vi "zadanie2pawelprokopiuk.vi"() -> ()   [LabVIEW 2021]
panel:
  out "min temp":dbl
  out "max temp":dbl
  in  "URL":string="dstp://10.42.14.239/temperatura"
  out "Temperatura":T1(graph)
  in  "stop":bool
  in  "Zapis do pliku":bool
  in  "prog dolny":dbl
  in  "prog gorny":dbl=25.8
  out "alarm dolny":bool
  out "alarm gorny":bool
  out "T chwilowa":dbl
  out "T srednia":dbl
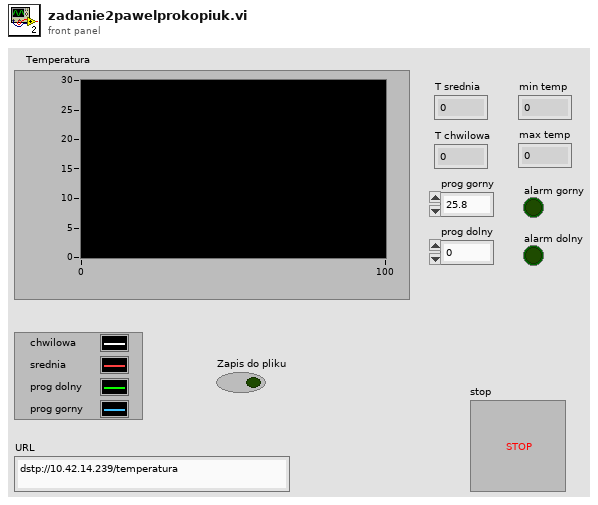
[diagram p1: front panel]
types:
  T1 = cluster{dbl, dbl, "Próg dolny":dbl, "Próg górny":dbl}
  T2 = enum16{"Read", "Write", "ReadWrite", "BufferedRead", "BufferedReadWrite"}
  T3 = enum16{"open", "replace", "create", "open or create", "replace or create", "replace or create with confirmation"}
  T4 = cluster{dbl, dbl, "prog dolny":dbl, "prog gorny":dbl}
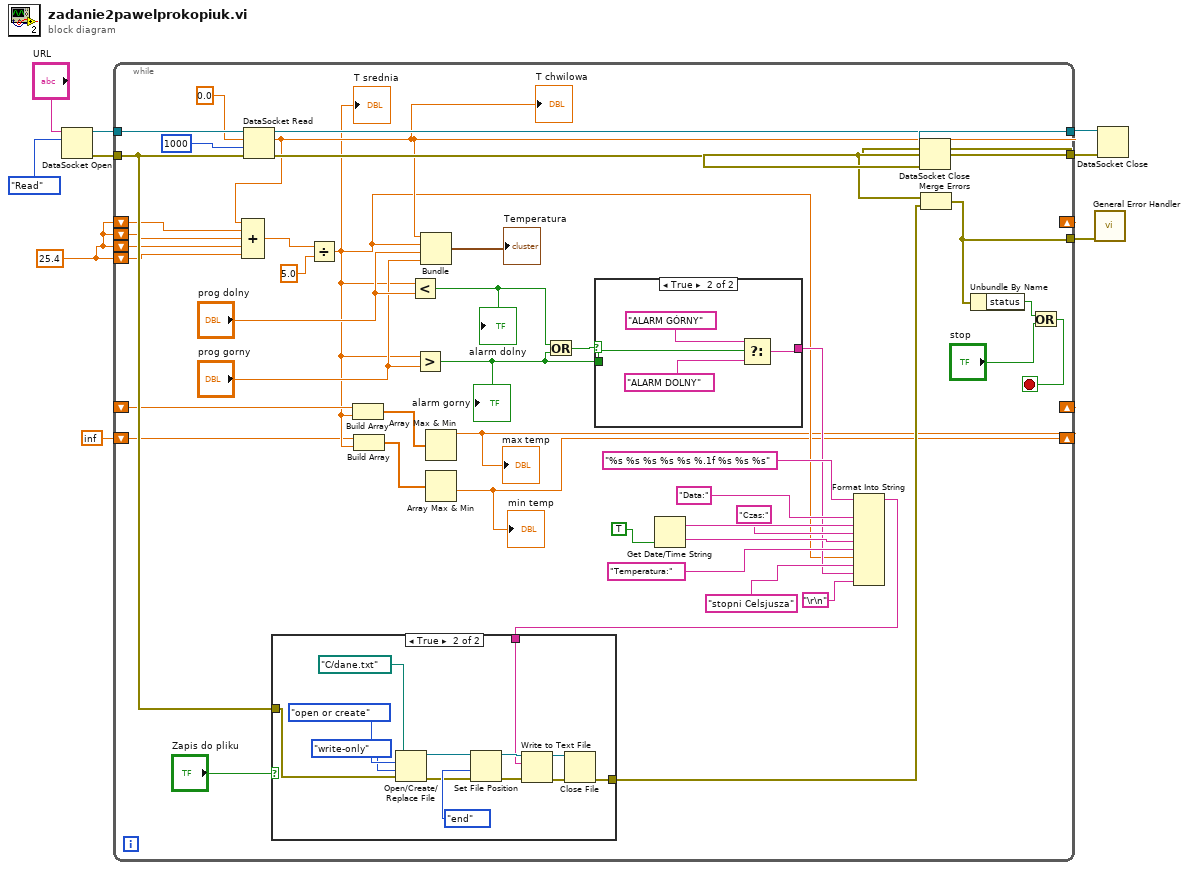
[diagram p0: block diagram]
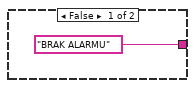
[diagram p2: hidden frame]
diagram:
  w2 = 25.4
  n1 = DataSocket Open(10:T2."Read" ("mode"), 11:"URL") -> (0:w8:errorcluster, 3:w9:refnum<k13>)  [unwired: 2 in]
  n2 = while {
    tunnel: w9 -> [w51]
    tunnel: [w50] -> w4
    tunnel: w8 -> [w44]
    tunnel: [w23] -> w3
    tunnel: [w42] -> w6
    shift-right: [w18] -> _
    shift-left: w2 -> [w22]
    shift-left: w2 -> [w21]
    shift-left: w2 -> [w20]
    shift-left: w2 -> [w19]
    shift-right: [w12] -> _
    shift-left: _ -> [w16]
    shift-right: [w11] -> _
    shift-left: inf -> [w14]
    stop <- w48 stop-if-true
    n3 = DataSocket Read(8:w44, 9:1000, 10:0.0, 11:w51) -> (0:w23:errorcluster, 2:w18:dbl, 3:w50:refnum<k13>)  [unwired: 1 in, 4 out]
    "T chwilowa" <- w18
    n4 = Compound Arithmetic op=ADD(w18, w22, w21, w20, w19) -> (w17:dbl)
    n5 = Divide(x=w17, y=5.0 ("x/y")) -> (x/y=w15:dbl)
    "T srednia" <- w15
    n6 = Build Array(w16, w15) -> (w13:dbl[])
    n7 = Build Array(w14, w15) -> (w10:dbl[])
    n8 = Less?(x=w15, y="prog dolny") -> (x < y?=w28:bool)
    "alarm dolny" <- w28
    n9 = Greater?(x=w15, y="prog gorny") -> (0:w25:bool)
    "alarm gorny" <- w25
    n10 = Bundle(w18, w15, "prog dolny"="prog dolny", "prog gorny"="prog gorny") -> (→"Temperatura":T4)  [unwired: 1 in]
    n11 = Array Max & Min(array=w13) -> (max value=w12:dbl)  [unwired: 3 out]
    "max temp" <- w12
    n12 = Array Max & Min(array=w10) -> (min value=w11:dbl)  [unwired: 3 out]
    "min temp" <- w11
    n13 = Or(x=w28, y=w25) -> (x .or. y?=w27:bool)
    n14 = case shown="True" w27 {
      tunnel: ["BRAK ALARMU" w55] -> w26
      tunnel: w25 -> [_ w54]
      frame False {
      }
      frame True {
        n15 = Select(t="ALARM GÓRNY", s=w54, f="ALARM DOLNY") -> (s? t:f=w55:string)
      }
    }
    n16 = Get Date/Time String(want seconds? (F)=TRUE) -> (date string=w39:string, time string=w37:string)  [unwired: 2 in]
    n17 = Format Into String(format string="%s %s %s %s %s %.1f %s %s %s", "Data:", w39, "Czas:", w37, "Temperatura:", w15, "stopni Celsjusza", w26, "\r\n") -> (resulting string=w24:string)  [unwired: 2 in, 1 out]
    n18 = case shown="True" "Zapis do pliku" {
      tunnel: w44 -> [w58 w66]
      tunnel: [w58 w62] -> w43
      tunnel: w24 -> [_ w59]
      frame False {
      }
      frame True {
        n19 = Open/Create/Replace File(file path (use dialog)=path "C:/dane.txt", error in=w66, operation (0:open)=T3."open or create", access (0:read/write)=enum16{"read/write", "read-only", "write-only"}."write-only") -> (refnum out=w64:refnum<file>, error out=w65:errorcluster)  [unwired: 2 in, 1 out]
        n20 = Set File Position(refnum=w64, from (0:start)=enum16{"start", "end", "current"}."end", error in=w65) -> (refnum out=w67:refnum<file>, error out=w68:errorcluster)  [unwired: 1 in]
        n21 = Write to Text File(file (use dialog)=w67, text=w59, error in=w68) -> (refnum out=w69:refnum<file>, error out=w70:errorcluster)  [unwired: 1 in, 1 out]
        n22 = Close File(refnum=w69, error in=w70) -> (error out=w62:errorcluster)  [unwired: 1 out]
      }
    }
    n23 = Merge Errors(w23, w43) -> (w42:errorcluster)
    n24 = Unbundle By Name(w42) -> ("status"=w49:bool)
    n25 = Or(x=w49, y="stop") -> (x .or. y?=w48:bool)
  }
  n26 = DataSocket Close(8:w3, 11:w4) -> ()  [unwired: 1 in, 2 out]
  n27 = call <vilib>:"General Error Handler.vi"("error in (no error)"=w6) -> ()  [unwired: 10 in, 5 out]
  n28 = DataSocket Close(8:w3, 11:w4) -> ()  [unwired: 1 in, 2 out]
